vi "Create.vi"(8 "error in (no error)":errorcluster, 9 "Loader Name":string, 10 "pid":u32, 11 "Plugin Manager in":refnum<class "CIFPluginLoader.lvclass">) -> (0 "error out":errorcluster, 3 "Plugin Manager out":refnum<class "CIFPluginLoader.lvclass">)   [LabVIEW 2021, in "CIFPluginLoader.lvclass"]
uses:
  CIFPluginLoader.lvclass
  CIFPluginLoader.lvclass/CIFPluginLoader.ctl
  CIFUtilities/CIFConfigurationFile/CIF Configuration File.lvlib
  CIFUtilities/CIFLogs/CIFLogs.lvlib
  CIFUtilities/CIFLogs/Typedef/Message Type.ctl
  typedef/Loaded Plugin Map.ctl
  CIFPluginManager/gRPC/CIF_Manager_Client_Wrapper/CIFManagerClientWrapper.lvlib
  CIFPluginManager/gRPC/CIF_Manager_client/RPC Messages/cif_manager_LoaderType.ctl
  CIFPluginManager/gRPC/CIF_Manager_client/CIF_Manager_client.lvlib
  CIFPluginManager/gRPC/CIF_Manager_client/RPC Messages/cif_manager_LoaderInfoFull.ctl
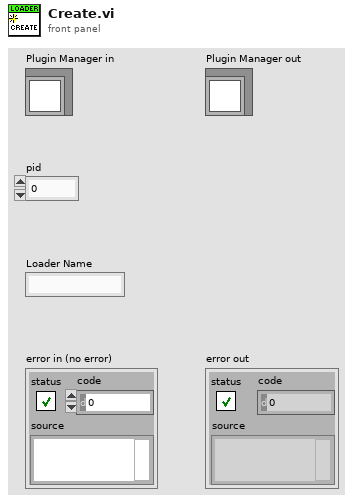
[diagram p1: front panel]
types:
  T1 = typedef "CIF_Manager_client.lvlib/cif_manager_LoaderType.ctl" = enum32{"LOADERTYPE_UNKNOWN", "LOADERTYPE_LABVIEW"}
  T2 = typedef "CIF_Manager_client.lvlib/cif_manager_LoaderInfoFull.ctl" = cluster{"loader_type":T1, "loader_name":string, "grpc_port":i32, "pid":u32}
  T3 = typedef "CIFPluginLoader.lvclass/Loaded Plugin Map.ctl" = map{string, refnum<vi>}
  T4 = typedef "CIFLogs.lvlib/Message Type.ctl" = enum16{"Error", "Information", "Print Terminal", "Configuration"}
  T5 = typedef "grpc-lvsupport-release.lvlib/grpcId.ctl" = u64
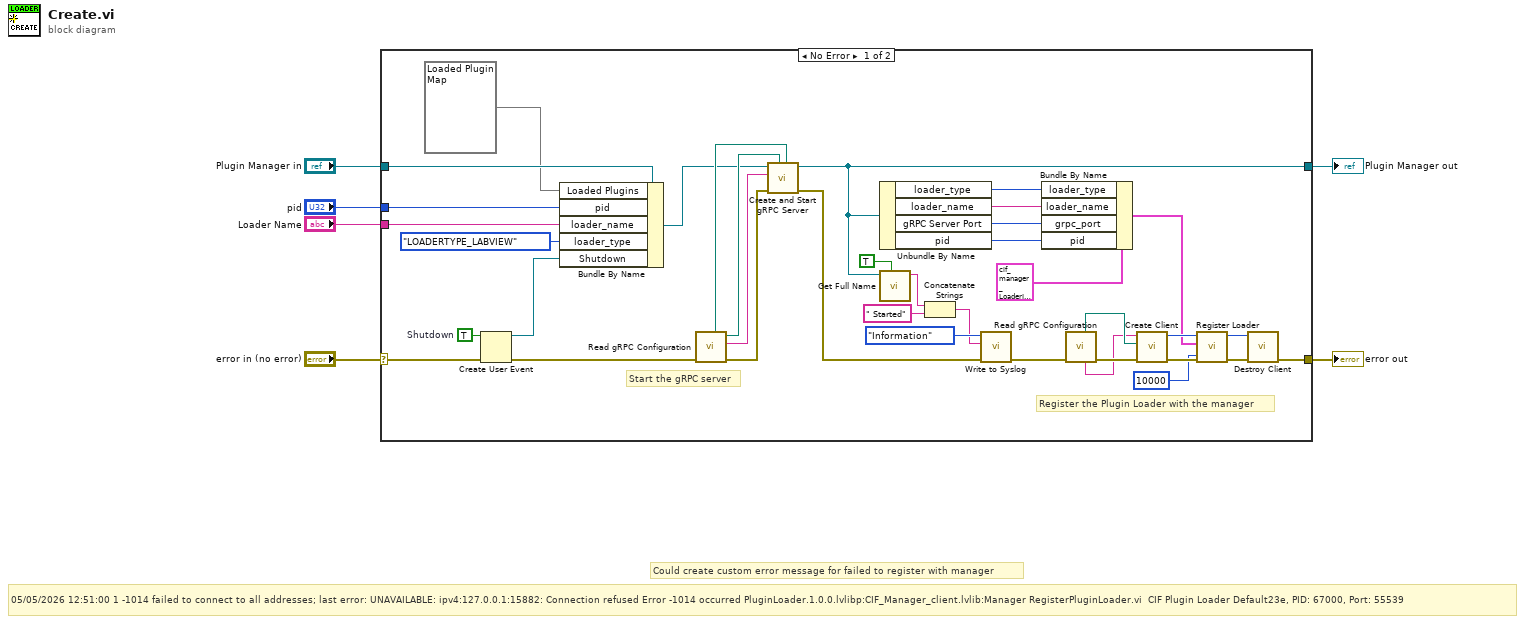
[diagram p0: block diagram]
diagram:
  # "05/05/2026 12:51:00\t1\t-1014\tfailed to connect to all addresses; last error: UNAVAILABLE: ipv4:127.0.0.1:15882: Connection refused\tError -1014 occurred PluginLoader.1.0.0.lvlibp:CIF_Manager_client.lvlib:Manager RegisterPluginLoader.vi \tCIF Plugin Loader Default23e, PID: 67000, Port: 55539"
  # "Could create custom error message for failed to register with manager"
  n1 = case shown="No Error" "error in (no error)" {
    selector: "error in (no error)" -> [w38 w45]
    tunnel: [w12 w45] -> w5
    tunnel: [w23 w44] -> w3
    tunnel: "Plugin Manager in" -> [w35 w44]
    tunnel: "pid" -> [w25 _]
    tunnel: "Loader Name" -> [w31 _]
    frame No Error {
      w39 = TRUE  # Shutdown
      # "Register the Plugin Loader with the manager"
      # "Start the gRPC server"
      n2 = Create User Event(user event datatype=w39, error in=w38) -> (user event=w33:refnum<user-event>, error out=w37:errorcluster)
      n3 = Bundle By Name(cluster=w35, "Loaded Plugins"=T3 {}, "pid"=w25, "loader_name"=w31, "loader_type"=cif_manager_LoaderType."LOADERTYPE_LABVIEW", "Shutdown"=w33) -> (w32:refnum<class "CIFPluginLoader.lvclass">)
      n4 = call "Read gRPC Configuration.vi"("error in"=w37) -> ("error out"=w43:errorcluster, "Plugin Server Address"=w26:string, "Server Certificate File (.crt)"=w41:path, "Server Key File (.key)"=w42:path)  [unwired: 5 in, 2 out]
      n5 = call "Create and Start gRPC Server.vi"("Server Key File (.key)"=w42, "Server Certificate File (.crt)"=w41, "error in (no error)"=w43, "Server Address"=w26, "CIFLauncher in"=w32) -> ("error out"=w36:errorcluster, "CIFLauncher out"=w23:refnum<class "CIFPluginLoader.lvclass">)  [unwired: 5 in]
      n6 = Unbundle By Name(w23) -> ("loader_type"=w9:T1, "loader_name"=w8:string, "gRPC Server Port"=w28:i32, "pid"=w27:u32)
      n7 = call "Get Full Name.vi"("Include Extra Info"=TRUE, "CIFPluginLoader in"=w23) -> ("Name"=w24:string)  [unwired: 9 in]
      n8 = Concatenate Strings(w24, " Started" ("message")) -> (w22:string)
      n9 = call "Write to Syslog.vi"("error in (no error)"=w36, "message"=w22, "CIF Message Type"=Message_Type."Information") -> ("error out"=w29:errorcluster)  [unwired: 8 in]
      n10 = Bundle By Name(cluster=T2 {"loader_type"=enum."LOADERTYPE_UNKNOWN", "loader_name"="", "grpc_port"=0, "pid"=0} ("Loader Info"), "loader_type"=w9, "loader_name"=w8, "grpc_port"=w28, "pid"=w27) -> (w20:T2)
      n11 = call "Read gRPC Configuration.vi"("error in"=w29) -> ("error out"=w15:errorcluster, "Local Manager Address"=w13:string, "Server Key File (.key)"=w14:path)  [unwired: 5 in, 3 out]
      n12 = call "Create Client.vi"("error in"=w15, "Server Certificate File (.crt)"=w14, "address"=w13) -> ("error out"=w19:errorcluster, "gRPC ID Out"=w21:T5)  [unwired: 7 in]
      n13 = call "Register Loader.vi"("timeout (ms)"=10000, "error in"=w19, "Loader Info"=w20, "gRPC ID in"=w21) -> ("error out"=w18:errorcluster, "gRPC ID out"=w17:T5)  [unwired: 6 in]
      n14 = call "Destroy Client.vi"("error in"=w18, "gRPC ID"=w17) -> ("error out"=w12:errorcluster)  [unwired: 9 in]
    }
    frame Error {
    }
  }
  "error out" <- w5
  "Plugin Manager out" <- w3
